vi "OAT Tachless Add Control Point.vi"(9 "chkpoint color":u32(colorbox)=15593216, 10 "Pop Pos":cluster{i32, i32}, 11 "Tracks Ref":refnum<vi>) -> ()   [LabVIEW 2017, in "SoundVib_Tachless.lvlib"]
uses:
  <vilib>/addons/Sound and Vibration/Order Analysis/Tachless/SoundVib_Tachless.lvlib
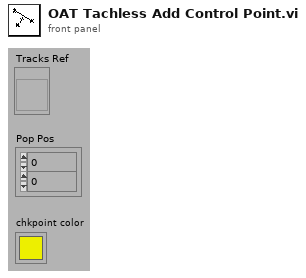
[diagram p1: front panel]
types:
  T1 = cluster{"Name":string, "Color":u32, "Style":u8, "Point Style":u8, "Name Visible":bool, "Allow Drag":bool, "Lock Style":u32, "Plot":u32, "Index":i32, "Position":cluster{"X":dbl, "Y":dbl}}[]
  T2 = cluster{"Name":string, "Color":u32, "Hair Style":u8, "Point Style":u8, "Name Visible":bool, "Trackable":bool, "Lock Style":u32, "Plot Number":u32, "Marker Index":i32, "Location":cluster{"X":dbl, "Y":dbl}}[]
  T3 = cluster{"Name":string, "Color":u32, "Hair Style":u8, "Point Style":u8, "Name Visible":bool, "Trackable":bool, "Lock Style":u32, "Plot Number":u32, "Marker Index":i32, "Location":cluster{"X":dbl, "Y":dbl}}
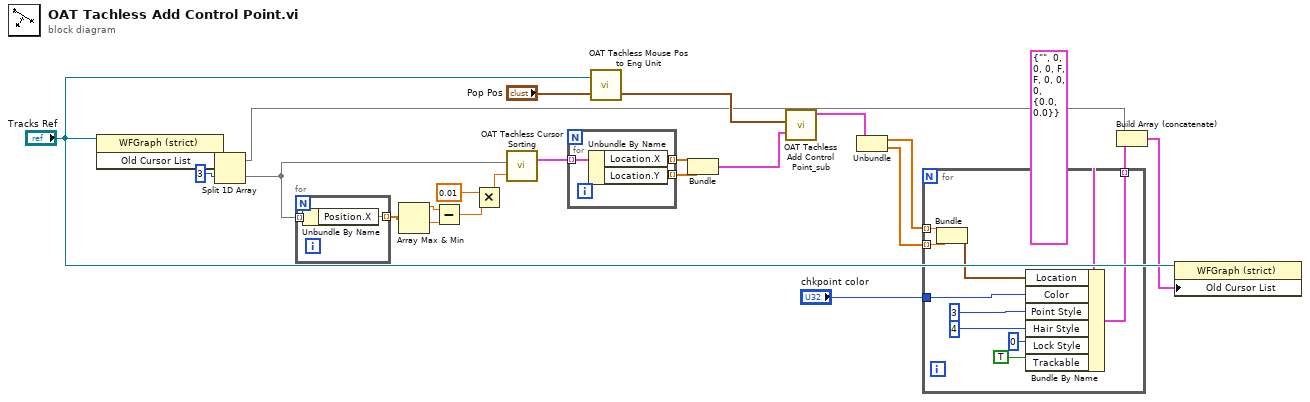
[diagram p0: block diagram]
diagram:
  n1 = property on="Property Node" class="WFGraph (strict)"(reference="Tracks Ref") -> ("Old Cursor List"=w15:T1)  [unwired: 1 in, 2 out]
  n2 = Split 1D Array(array=w15, index=3 ("Array Index")) -> (first subarray=w2:T1, second subarray=w1:T1)
  n3 = for {
    tunnel: w1 -> [w25] mode=indexing
    tunnel: [w24] -> w8 mode=indexing
    n4 = Unbundle By Name(w25) -> ("Position.X"=w24:dbl)
  }
  n5 = Array Max & Min(array=w8) -> (max value=w7:dbl, min value=w6:dbl)  [unwired: 2 out]
  n6 = Subtract(x=w7, y=w6) -> (x-y=w5:dbl)
  n7 = Multiply(x=0.01, y=w5) -> (x*y=w3:dbl)
  n8 = call <vilib>:"OAT Tachless Cursor Sorting.vi"("Numeric"=w3, "Array"=w1) -> ("Array 2"=w9:T2)
  n9 = for {
    tunnel: w9 -> [w28] mode=indexing
    tunnel: [w27] -> w13 mode=indexing
    tunnel: [w26] -> w14 mode=indexing
    n10 = Unbundle By Name(w28) -> ("Location.X"=w27:dbl, "Location.Y"=w26:dbl)
  }
  n11 = call <vilib>:"OAT Tachless Mouse Pos to Eng Unit.vi"("Pop Pos"="Pop Pos", "Tracks ref"="Tracks Ref") -> ("Control Point"=w11:cluster{dbl, dbl})  [unwired: 1 in]
  n12 = Bundle(w13, w14) -> (w21:cluster{dbl[], dbl[]})  [unwired: 1 in]
  n13 = call <vilib>:"OAT Tachless Add Control Point_sub.vi"("New Control Point"=w11, "Control Points"=w21) -> ("Control Points Out"=w22:cluster{"X":dbl[], "Y":dbl[]})  [unwired: 9 in]
  n14 = Unbundle(w22) -> ("X"=w17:dbl[], "Y"=w18:dbl[])
  n15 = for {
    tunnel: "chkpoint color" -> [w38]
    tunnel: w17 -> [w32] mode=indexing
    tunnel: w18 -> [w31] mode=indexing
    tunnel: [w29] -> w23 mode=indexing
    n16 = Bundle("Numeric"=w32, "Numeric"=w31) -> (w30:cluster{"Numeric":dbl, "Numeric":dbl})  [unwired: 1 in]
    n17 = Bundle By Name(cluster=T3 {"Name"="", "Color"=0, "Hair Style"=0, "Point Style"=0, "Name Visible"=FALSE, "Trackable"=FALSE, "Lock Style"=0, "Plot Number"=0, "Marker Index"=0, "Location"={"X"=0.0, "Y"=0.0}} ("Input Cluster"), "Location"=w30, "Color"=w38, "Point Style"=u8 3 ("Hair Style"), "Hair Style"=u8 4, "Lock Style"=u32 0, "Trackable"=TRUE) -> (w29:T3)
  }
  n18 = Build Array (concatenate)(w2, w23) -> (w19:T2)
  n19 = property on="Property Node" class="WFGraph (strict)"(reference="Tracks Ref", "Old Cursor List"=w19) -> ()  [unwired: 1 in, 2 out]
